vi "Add Timestamp to Waveforms.vi"(7 "initialize":bool, 10 "waveforms":waveform(dbl)[](array[waveform])) -> (2 "waveforms":waveform(dbl)[](array[waveform]))   [LabVIEW 2022 SP3]
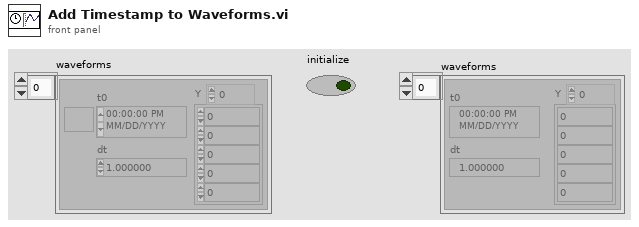
[diagram p1: front panel]
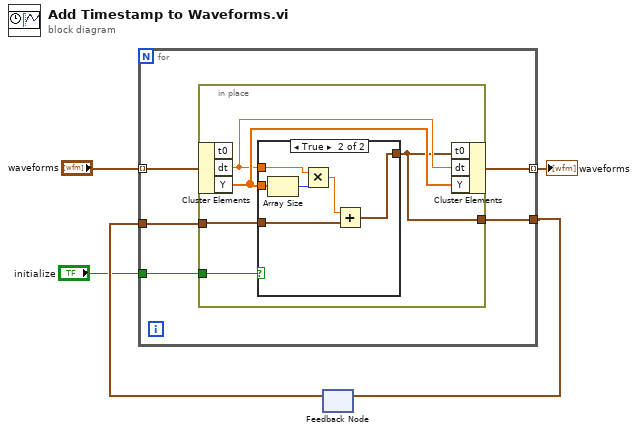
[diagram p0: block diagram]
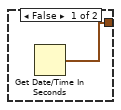
[diagram p2: hidden frame]
diagram:
  n1 = feedback #1() -> (w4:timestamp)  [unwired: 1 in]
  n2 = for {
    tunnel: "waveforms" -> [w10] mode=indexing
    tunnel: w4 -> [w9]
    tunnel: [w8] -> w3
    tunnel: "initialize" -> [w7]
    tunnel: [w6] -> w2 mode=indexing
    n3 = in-place {
      in-place-border: w9 -> [w15]
      in-place-border: [w11] -> w8
      in-place-border: w7 -> [w14]
      n4 = in-place-cluster #2(w10) -> ("dt"=w12:dbl, "Y"=w13:dbl[])  [unwired: 1 out]
      n5 = case shown="True" w14 {
        tunnel: w13 -> [_ w22]
        tunnel: w12 -> [_ w20]
        tunnel: w15 -> [_ w18]
        tunnel: [w16 w17] -> w11
        frame False {
          n6 = Get Date/Time In Seconds() -> (seconds since 1Jan1904=w16:timestamp)
        }
        frame True {
          n7 = Array Size(array=w22) -> (size(s)=w21:i32)
          n8 = Multiply(x=w20, y=w21) -> (x*y=w19:dbl)
          n9 = Add(x=w19, y=w18) -> (x+y=w17:timestamp)
        }
      }
      n10 = in-place-cluster #2("t0"=w11, "dt"=w12, "Y"=w13) -> (w6:waveform(dbl))
    }
  }
  "waveforms" <- w2
  n11 = feedback-in #1(w3) -> ()
